vi "GetFtpCurrentPosition.vi"(10 "Ftp":refnum<k24>, 11 "error in":errorcluster) -> (2 "Current position":T1(array[cluster]), 3 "error out":errorcluster)   [LabVIEW 2018, in "UnderAutomation.Fanuc.lvlib"]
uses:
  UnderAutomation.Fanuc.lvlib
  C:/Users/fg/Documents/Fanuc.vi/LabVIEW_2024/UnderAutomation.Fanuc/lib/UnderAutomation.Fanuc.dll
  LabVIEW_2024/UnderAutomation.Fanuc/lib/UnderAutomation.Fanuc.dll
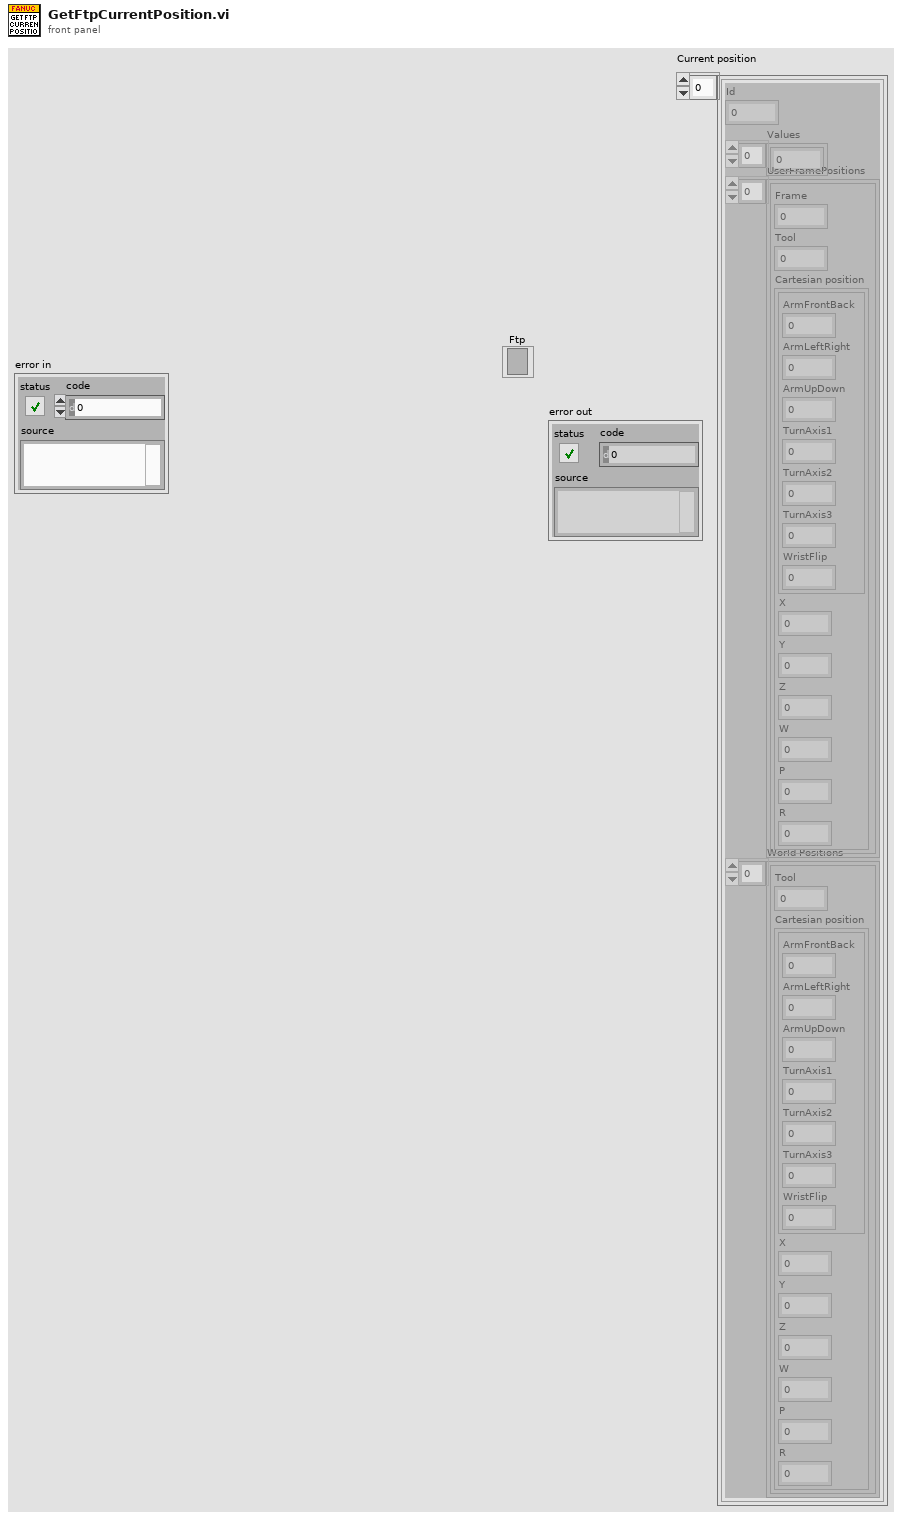
[diagram p1: front panel]
types:
  T1 = cluster{"Id":i32, "Values":dbl[], "UserFramePositions":cluster{"Frame":i32, "Tool":i32, "Cartesian position":cluster{cluster{"ArmFrontBack":i32, "ArmLeftRight":i32, "ArmUpDown":i32, "TurnAxis1":i32, "TurnAxis2":i32, "TurnAxis3":i32, "WristFlip":i32}, "X":dbl, "Y":dbl, "Z":dbl, "W":dbl, "P":dbl, "R":dbl}}[], "World Positions":cluster{"Tool":i32, "Cartesian position":cluster{cluster{"ArmFrontBack":i32, "ArmLeftRight":i32, "ArmUpDown":i32, "TurnAxis1":i32, "TurnAxis2":i32, "TurnAxis3":i32, "WristFlip":i32}, "X":dbl, "Y":dbl, "Z":dbl, "W":dbl, "P":dbl, "R":dbl}}[]}[]
  T2 = cluster{"Configuration":cluster{"ArmFrontBack":i32, "ArmLeftRight":i32, "ArmUpDown":i32, "TurnAxis1":i32, "TurnAxis2":i32, "TurnAxis3":i32, "WristFlip":i32}, "X":dbl, "Y":dbl, "Z":dbl, "W":dbl, "P":dbl, "R":dbl}
  T3 = cluster{"Frame":i32, "Tool":i32, "Cartesian position":cluster{"Configuration":cluster{"ArmFrontBack":i32, "ArmLeftRight":i32, "ArmUpDown":i32, "TurnAxis1":i32, "TurnAxis2":i32, "TurnAxis3":i32, "WristFlip":i32}, "X":dbl, "Y":dbl, "Z":dbl, "W":dbl, "P":dbl, "R":dbl}}
  T4 = cluster{"Tool":i32, "Cartesian position":cluster{"Configuration":cluster{"ArmFrontBack":i32, "ArmLeftRight":i32, "ArmUpDown":i32, "TurnAxis1":i32, "TurnAxis2":i32, "TurnAxis3":i32, "WristFlip":i32}, "X":dbl, "Y":dbl, "Z":dbl, "W":dbl, "P":dbl, "R":dbl}}
  T5 = cluster{"Id":i32, "Values":dbl[], cluster{"Frame":i32, "Tool":i32, "Cartesian position":cluster{"Configuration":cluster{"ArmFrontBack":i32, "ArmLeftRight":i32, "ArmUpDown":i32, "TurnAxis1":i32, "TurnAxis2":i32, "TurnAxis3":i32, "WristFlip":i32}, "X":dbl, "Y":dbl, "Z":dbl, "W":dbl, "P":dbl, "R":dbl}}[], cluster{"Tool":i32, "Cartesian position":cluster{"Configuration":cluster{"ArmFrontBack":i32, "ArmLeftRight":i32, "ArmUpDown":i32, "TurnAxis1":i32, "TurnAxis2":i32, "TurnAxis3":i32, "WristFlip":i32}, "X":dbl, "Y":dbl, "Z":dbl, "W":dbl, "P":dbl, "R":dbl}}[]}
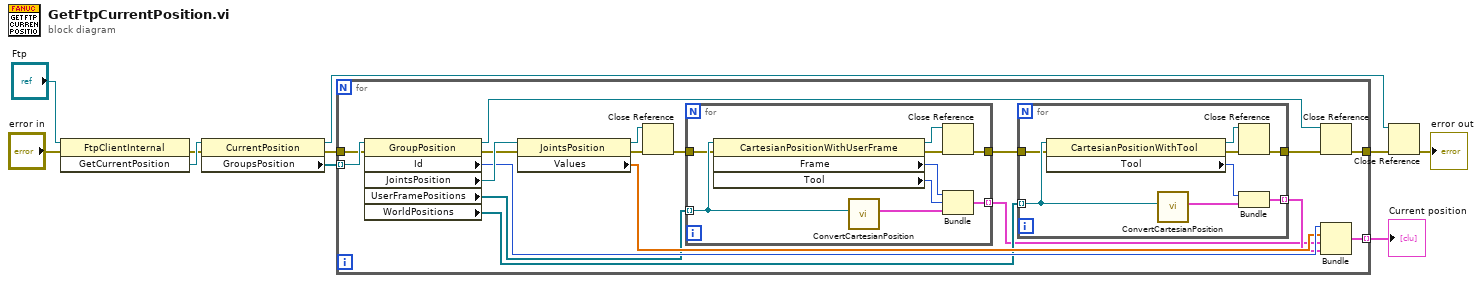
[diagram p0: block diagram]
diagram:
  n1 = invoke class="FtpClientInternal" method="GetCurrentPosition"(reference="Ftp", error in="error in") -> (error out=w3:errorcluster, "GetCurrentPosition"=w8:refnum<k24>)  [unwired: 1 in, 1 out]
  n2 = property class="CurrentPosition"(reference=w8, error in=w3) -> (reference out=w5:refnum<k24>, error out=w2:errorcluster, "GroupsPosition"=w7:refnum<k24>[])
  n3 = for {
    tunnel: w7 -> [w28] mode=indexing
    tunnel: [w21] -> w6 mode=indexing
    tunnel: [w13] -> w4
    tunnel: w2 -> [w12]
    n4 = property class="GroupPosition"(reference=w28, error in=w12) -> (reference out=w17:refnum<k24>, error out=w18:errorcluster, "Id"=w26:i32, "JointsPosition"=w27:refnum<k24>, "UserFramePositions"=w24:refnum<k24>[], "WorldPositions"=w23:refnum<k24>[])
    n5 = property class="JointsPosition"(reference=w27, error in=w18) -> (reference out=w20:refnum<k24>, error out=w19:errorcluster, "Values"=w25:dbl[])
    n6 = Close Reference(reference=w20, error in (no error)=w19) -> (error out=w11:errorcluster)
    n7 = for {
      tunnel: w24 -> [w43] mode=indexing
      tunnel: [w41] -> w16 mode=indexing
      tunnel: [w38] -> w15
      tunnel: w11 -> [w37]
      n8 = property class="CartesianPositionWithUserFrame"(reference=w43, error in=w37) -> (reference out=w40:refnum<k24>, error out=w39:errorcluster, "Frame"=w45:i32, "Tool"=w44:i32)
      n9 = call "ConvertCartesianPosition.vi"("Cartesian position"=w43) -> ("Cartesian position"=w42:T2)  [unwired: 9 in, 1 out]
      n10 = Close Reference(reference=w40, error in (no error)=w39) -> (error out=w38:errorcluster)
      n11 = Bundle("Frame"=w45, "Tool"=w44, "Cartesian position"=w42) -> (w41:T3)  [unwired: 1 in]
    }
    n12 = for {
      tunnel: w23 -> [w34] mode=indexing
      tunnel: [w29] -> w22 mode=indexing
      tunnel: w15 -> [w31]
      tunnel: [w30] -> w14
      n13 = property class="CartesianPositionWithTool"(reference=w34, error in=w31) -> (reference out=w33:refnum<k24>, error out=w32:errorcluster, "Tool"=w36:i32)
      n14 = call "ConvertCartesianPosition.vi"("Cartesian position"=w34) -> ("Cartesian position"=w35:T2)  [unwired: 9 in, 1 out]
      n15 = Close Reference(reference=w33, error in (no error)=w32) -> (error out=w30:errorcluster)
      n16 = Bundle("Tool"=w36, "Cartesian position"=w35) -> (w29:T4)  [unwired: 1 in]
    }
    n17 = Close Reference(reference=w17, error in (no error)=w14) -> (error out=w13:errorcluster)
    n18 = Bundle("Id"=w26, "Values"=w25, w16, w22) -> (w21:T5)  [unwired: 1 in]
  }
  "Current position" <- w6
  n19 = Close Reference(reference=w5, error in (no error)=w4) -> (error out=→"error out":errorcluster)
